vi "Style--constant.vi"() -> (3 "Style":T1={"Gris Obscuro Azul"=4079166, "Gris Medio Azul"=9343126, "Gris Claro Azul"=13817819, "Amarillo"=16763904, "Text color"=4079166, "Transparent"=4079166, "Fuente"="", "Text.Font:Size"=15})   [LabVIEW 2020, in "ConstantErrorsMaker.lvlib"]
uses:
  ConstantErrorsMaker.lvlib
  Style--cluster.ctl
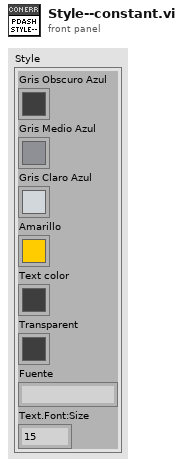
[diagram p1: front panel]
types:
  T1 = typedef "ConstantErrorsMaker.lvlib/Style--cluster.ctl" = cluster{"Gris Obscuro Azul":u32, "Gris Medio Azul":u32, "Gris Claro Azul":u32, "Amarillo":u32, "Text color":u32, "Transparent":u32, "Fuente":string, "Text.Font:Size":u32}
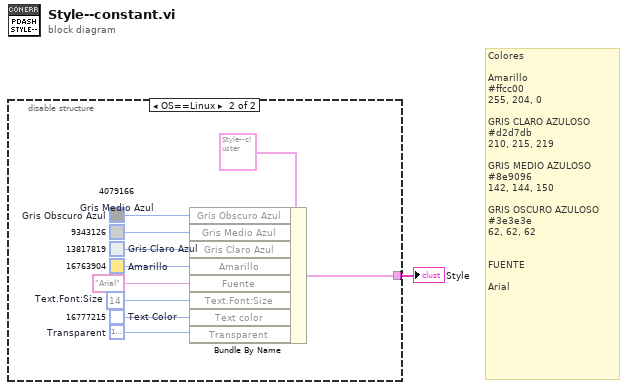
[diagram p0: block diagram]
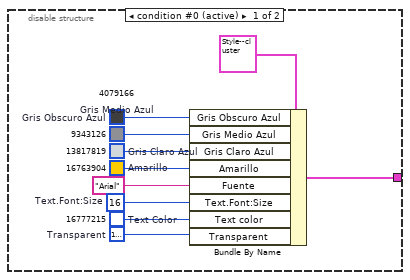
[diagram p2: hidden frame]
diagram:
  # "Colores\n\nAmarillo\n#ffcc00\n255, 204, 0\n\nGRIS CLARO AZULOSO\n#d2d7db\n210, 215, 219\n\nGRIS MEDIO AZULOSO\n#8e9096\n142, 144, 150\n\nGRIS OSCURO AZULOSO\n#3e3e3e\n62, 62, 62\n\n\nFUENTE\n\nArial"
  n1 = disable-structure shown="OS==Linux" {
    disable-tunnel: [w2 w12] -> w1
    frame condition #0 (active) {
      w3 = u32 16777216  # Transparent
      w4 = u32 16777215  # Text Color
      w5 = u32 16  # Text.Font:Size
      w7 = u32 16763904  # Amarillo
      w8 = u32 13817819  # Gris Claro Azul
      w9 = u32 9343126  # Gris Medio Azul
      w10 = u32 4079166  # Gris Obscuro Azul
      n2 = Bundle By Name(cluster=T1 {"Gris Obscuro Azul"=4079166, "Gris Medio Azul"=9343126, "Gris Claro Azul"=13817819, "Amarillo"=16763904, "Text color"=4079166, "Transparent"=4079166, "Fuente"="", "Text.Font:Size"=15}, "Gris Obscuro Azul"=w10, "Gris Medio Azul"=w9, "Gris Claro Azul"=w8, "Amarillo"=w7, "Fuente"="Arial", "Text.Font:Size"=w5, "Text color"=w4, "Transparent"=w3) -> (w2:T1)
    }
    frame condition #1 {
      w13 = u32 16777216  # Transparent
      w14 = u32 16777215  # Text Color
      w15 = u32 14  # Text.Font:Size
      w17 = u32 16763904  # Amarillo
      w18 = u32 13817819  # Gris Claro Azul
      w19 = u32 9343126  # Gris Medio Azul
      w20 = u32 4079166  # Gris Obscuro Azul
      n3 = Bundle By Name(cluster=T1 {"Gris Obscuro Azul"=4079166, "Gris Medio Azul"=9343126, "Gris Claro Azul"=13817819, "Amarillo"=16763904, "Text color"=4079166, "Transparent"=4079166, "Fuente"="", "Text.Font:Size"=15}, "Gris Obscuro Azul"=w20, "Gris Medio Azul"=w19, "Gris Claro Azul"=w18, "Amarillo"=w17, "Fuente"="Arial", "Text.Font:Size"=w15, "Text color"=w14, "Transparent"=w13) -> (w12:T1)
    }
  }
  "Style" <- w1
